vi "ULx Write (Analog Wfm 1Chan 1Samp).vi"(0 "task in":refnum<k24>, 1 "auto start":bool=TRUE, 7 "data":waveform(dbl)={"t0"=timestamp(0 s since 1904-01-01), "dt"=0.0, "Y"=[]}, 9 "timeout":dbl=10.0 format="%_4g", 11 "error in":errorcluster) -> (4 "task out":refnum<k24>, 10 "number of samples written per channel":u32, 15 "error out":errorcluster)   [LabVIEW 2020]
doc: "Writes a waveform that contains a single sample to a task that contains a single analog output channel."
uses:
  C:/Users/William/Documents/LV 2020 builds/LeaktestDAQ/Source-v33/ULx_LV.dll
  ULx_LV.dll
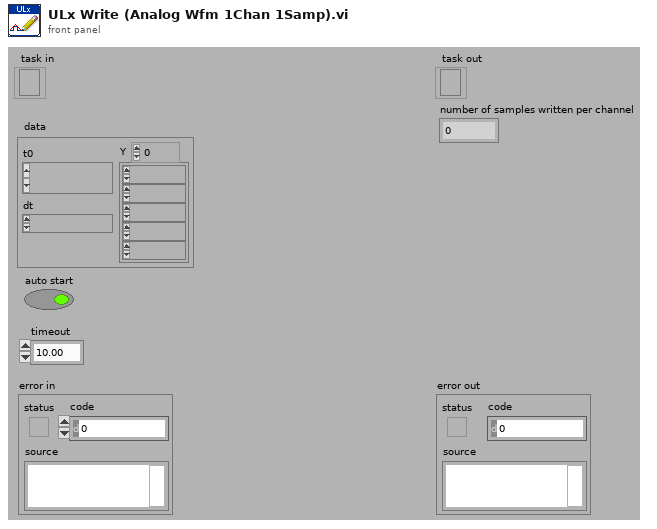
[diagram p1: front panel]
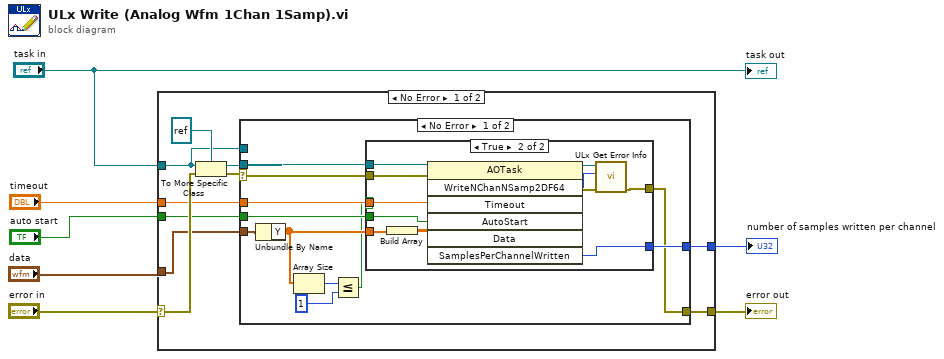
[diagram p0: block diagram]
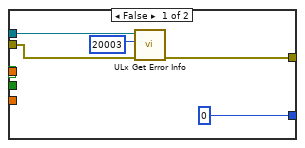
[diagram p2: hidden frame]
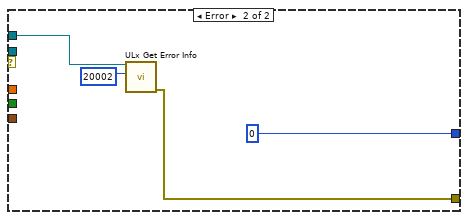
[diagram p3: hidden frame]
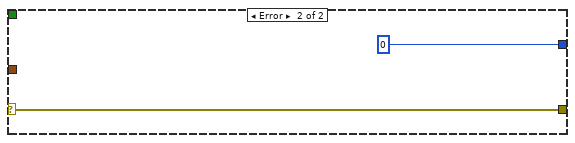
[diagram p4: hidden frame]
diagram:
  n1 = case shown="No Error" "error in" {
    selector: "error in" -> [w17 w50]
    tunnel: "task in" -> [w11 _]
    tunnel: "timeout" -> [w13 _]
    tunnel: [w12 w50] -> w5
    tunnel: "auto start" -> [w10 _]
    tunnel: [w9 0 ("SamplesPerChannelWritten")] -> w2
    tunnel: "data" -> [w8 _]
    frame No Error {
      n2 = To More Specific Class(target class=refnum<k24> refnum, reference=w11, error in=w17) -> (specific class reference=w14:refnum<k24>, error out=w15:errorcluster)
      n3 = case shown="No Error" w15 {
        selector: w15 -> [w27 _]
        tunnel: w14 -> [w28 _]
        tunnel: w13 -> [w25 _]
        tunnel: [w18 w47] -> w12
        tunnel: w11 -> [_ w46]
        tunnel: w10 -> [w24 _]
        tunnel: [w26 0 ("SamplesPerChannelWritten")] -> w9
        tunnel: w8 -> [w23 _]
        frame No Error {
          n4 = Unbundle By Name(w23) -> ("Y"=w22:dbl[])
          n5 = Array Size(array=w22) -> (size(s)=w21:i32)
          n6 = Less Or Equal?(x=w21, y=1) -> (x <= y?=w19:bool)
          n7 = case shown="True" w19 {
            tunnel: w28 -> [w31 w44]
            tunnel: w27 -> [w32 w43]
            tunnel: [u32 0 ("SamplesPerChannelWritten") w39] -> w26
            tunnel: w25 -> [_ w38]
            tunnel: w24 -> [_ w37]
            tunnel: w22 -> [_ w35]
            tunnel: [w33 w36] -> w18
            frame False {
              n8 = call "ULx Get Error Info.vi"("error in"=w32, "ErrorCode"=20003, "task in"=w31) -> ("error out"=w33:errorcluster)  [unwired: 8 in]
            }
            frame True {
              n9 = Build Array(w35) -> (w34:dbl[][])
              n10 = invoke class="AOTask" method="WriteNChanNSamp2DF64"(reference=w44, error in=w43, "Timeout"=w38, "AutoStart"=w37, "Data"=w34) -> (reference out=w41:refnum<k24>, error out=w42:errorcluster, "WriteNChanNSamp2DF64"=w40:i32, "SamplesPerChannelWritten"=w39:u32)  [unwired: 2 in, 3 out]
              n11 = call "ULx Get Error Info.vi"("error in"=w42, "ErrorCode"=w40, "task in"=w41) -> ("error out"=w36:errorcluster)  [unwired: 8 in]
            }
          }
        }
        frame Error {
          n12 = call "ULx Get Error Info.vi"("ErrorCode"=20002, "task in"=w46) -> ("error out"=w47:errorcluster)  [unwired: 9 in]
        }
      }
    }
    frame Error {
    }
  }
  "error out" <- w5
  "number of samples written per channel" <- w2
  "task out" <- "task in"
